vi "create_data_folders.vi"(9 "Experiment Title":string, 10 "Username":string, 11 "Folderpath on C:":path) -> (3 "Folderpath on C: out":path)   [LabVIEW 2018]
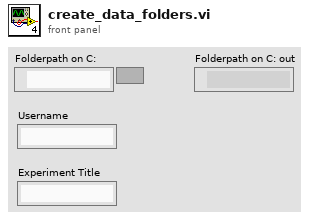
[diagram p1: front panel]
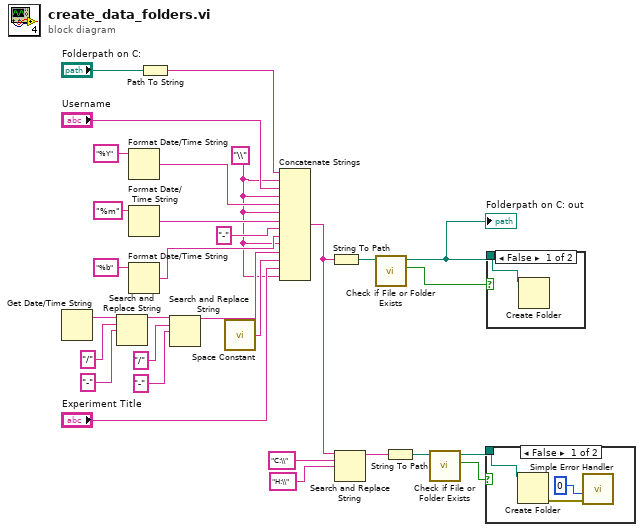
[diagram p0: block diagram]
diagram:
  w3 = "\\"
  n1 = Get Date/Time String() -> (date string=w18:string)  [unwired: 3 in, 1 out]
  n2 = Search and Replace String(input string=w18, search string="/", replace string="-") -> (result string=w26:string)  [unwired: 5 in, 3 out]
  n3 = Format Date/Time String(time format string (%c)="%Y") -> (date/time string=w11:string)  [unwired: 2 in]
  n4 = Format Date/Time String(time format string (%c)="%m") -> (date/time string=w12:string)  [unwired: 2 in]
  n5 = Format Date/Time String(time format string (%c)="%b") -> (date/time string=w13:string)  [unwired: 2 in]
  n6 = Path To String(path="Folderpath on C:") -> (string=w1:string)
  n7 = Search and Replace String(input string=w26, search string="/", replace string="-") -> (result string=w27:string)  [unwired: 5 in, 3 out]
  n8 = call <vilib>:"Space Constant.vi"() -> ("String"=w28:string)
  n9 = Concatenate Strings(w1, w3, "Username", w3, w11, w3, w12, "-", w13, w3, w27, w28, "Experiment Title", w3) -> (w30:string)
  n10 = String To Path(string=w30) -> (path=w6:path)
  n11 = Search and Replace String(input string=w30, search string="C:\\", replace string="H:\\") -> (result string=w21:string)  [unwired: 5 in, 3 out]
  n12 = call <vilib>:"Check if File or Folder Exists.vi"("path"=w6) -> ("file or folder exists?"=w5:bool, "dup path"=w4:path)  [unwired: 8 in, 1 out]
  "Folderpath on C: out" <- w4
  n13 = String To Path(string=w21) -> (path=w17:path)
  n14 = call <vilib>:"Check if File or Folder Exists.vi"("path"=w17) -> ("file or folder exists?"=w16:bool, "dup path"=w15:path)  [unwired: 8 in, 1 out]
  n15 = case shown="False" w16 {
    tunnel: w15 -> [w33 _]
    frame False {
      n16 = Create Folder(path (use dialog)=w33) -> (error out=w32:errorcluster)  [unwired: 2 in, 2 out]
      n17 = call <vilib>:"Simple Error Handler.vi"("type of dialog (OK msg:1)"=0, "error in (no error)"=w32) -> ()  [unwired: 3 in, 5 out]
    }
    frame True {
    }
  }
  n18 = case shown="False" w5 {
    tunnel: w4 -> [w34 _]
    frame False {
      n19 = Create Folder(path (use dialog)=w34) -> ()  [unwired: 2 in, 3 out]
    }
    frame True {
    }
  }
